vi "MicroGridExample.vi"() -> ()   [LabVIEW 2018]
uses:
  <vilib>/OPCUA/controls/NodeIds.ctl
  <vilib>/OPCUA/controls/NodeId.ctl
  <vilib>/OPCUA/client/Multiple Read Variant.vi
  GlobalVal.vi
  <vilib>/OPCUA/NI OPC UA Client.lvlib
panel:
  out "timestamp":timestamp
  out "OPCUA Server Error Log":errorcluster
  in  "Connect to Main Grid":bool
  out "Slide 8":u8(slide)
  out "Slide 7":u8(slide)
  out "Slide 6":u8(slide)
  out "Slide 5":u8(slide)
  out "Slide 4":u8(slide)
  out "Slide 2":u8(slide)
  out "Slide":u8(slide) scale=0.0..100.0
  out "Slide 3":u8(slide) scale=0.0..100.0
  out "Power":u8(slide) scale=0.0..100.0
  out "Power":u8(slide) scale=0.0..100.0
  in  "Tank":dbl(slide) scale=0.0..10.0
  in  "Photovoltaic":bool
  in  "Battery":bool
  out "Power":u8(slide) scale=0.0..100.0
  out "Power":u8(slide) scale=0.0..100.0
  out "Ki":dbl
  out "Kp":dbl
  out "tP":dbl
  out "kP":dbl
  in  "kP":dbl step=0.1
  in  "tf":dbl step=0.1
  out "tf":dbl
  out "kf":dbl
  in  "kf":dbl step=0.1
  in  "Ki":dbl step=0.1
  in  "Kp":dbl step=0.1
  in  "tP":dbl step=0.1
  in  "Program Stop":bool
  in  "Disconnect":bool
  in  "Connect Server":bool
  in  "OPC Server URL":string
  in  "Diesel 2":bool
  in  "Diesel 1":bool
  out "Device":string="PowerGenerator"
  in  "Solar irradiance":dbl(knob) scale=0.0..10.0
  in  "Load power":dbl(knob) scale=0.0..10.0
  in  "stop":bool
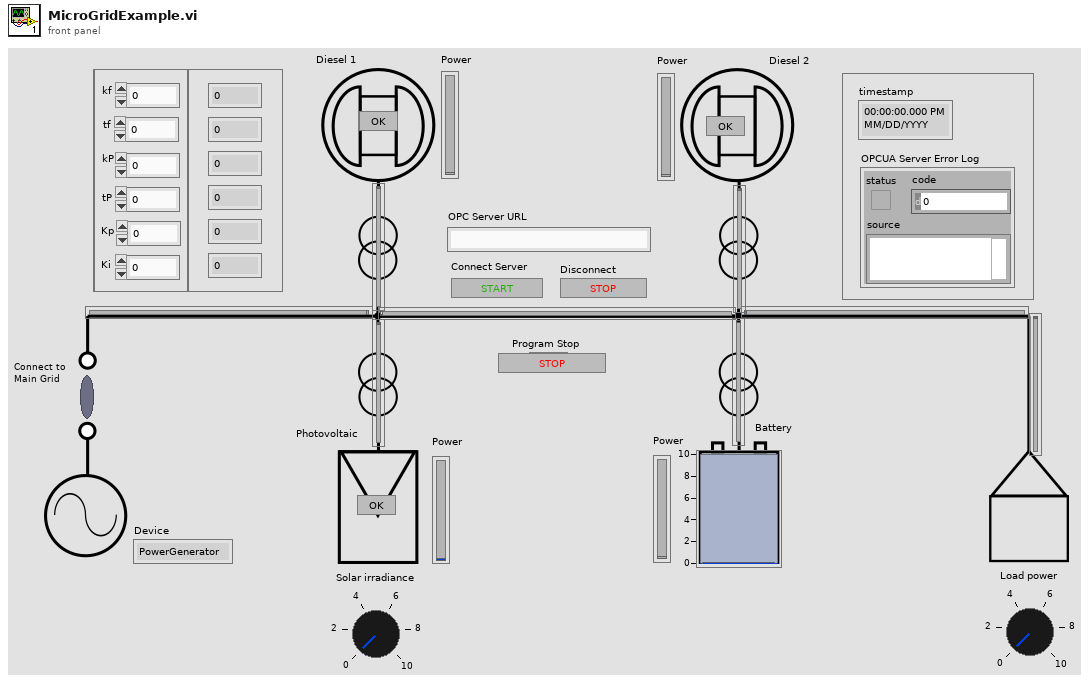
[diagram p1: front panel]
types:
  T1 = typedef "NodeIds.ctl" = T2[]
  T2 = typedef "NodeId.ctl" = string
  T3 = typedef "OPC UA Client Refnum.ctl" = refnum<k21>
  T4 = typedef "Read Variant Result.ctl" = cluster{"node ID":T2, "value ":variant, "timestamp":timestamp, "status":T5}
  T5 = typedef "OPC UA StatusCode.ctl" = u32
  T6 = enum32{"Invalid", "Standard", "Closed", "Hidden", "Minimized", "Maximized"}
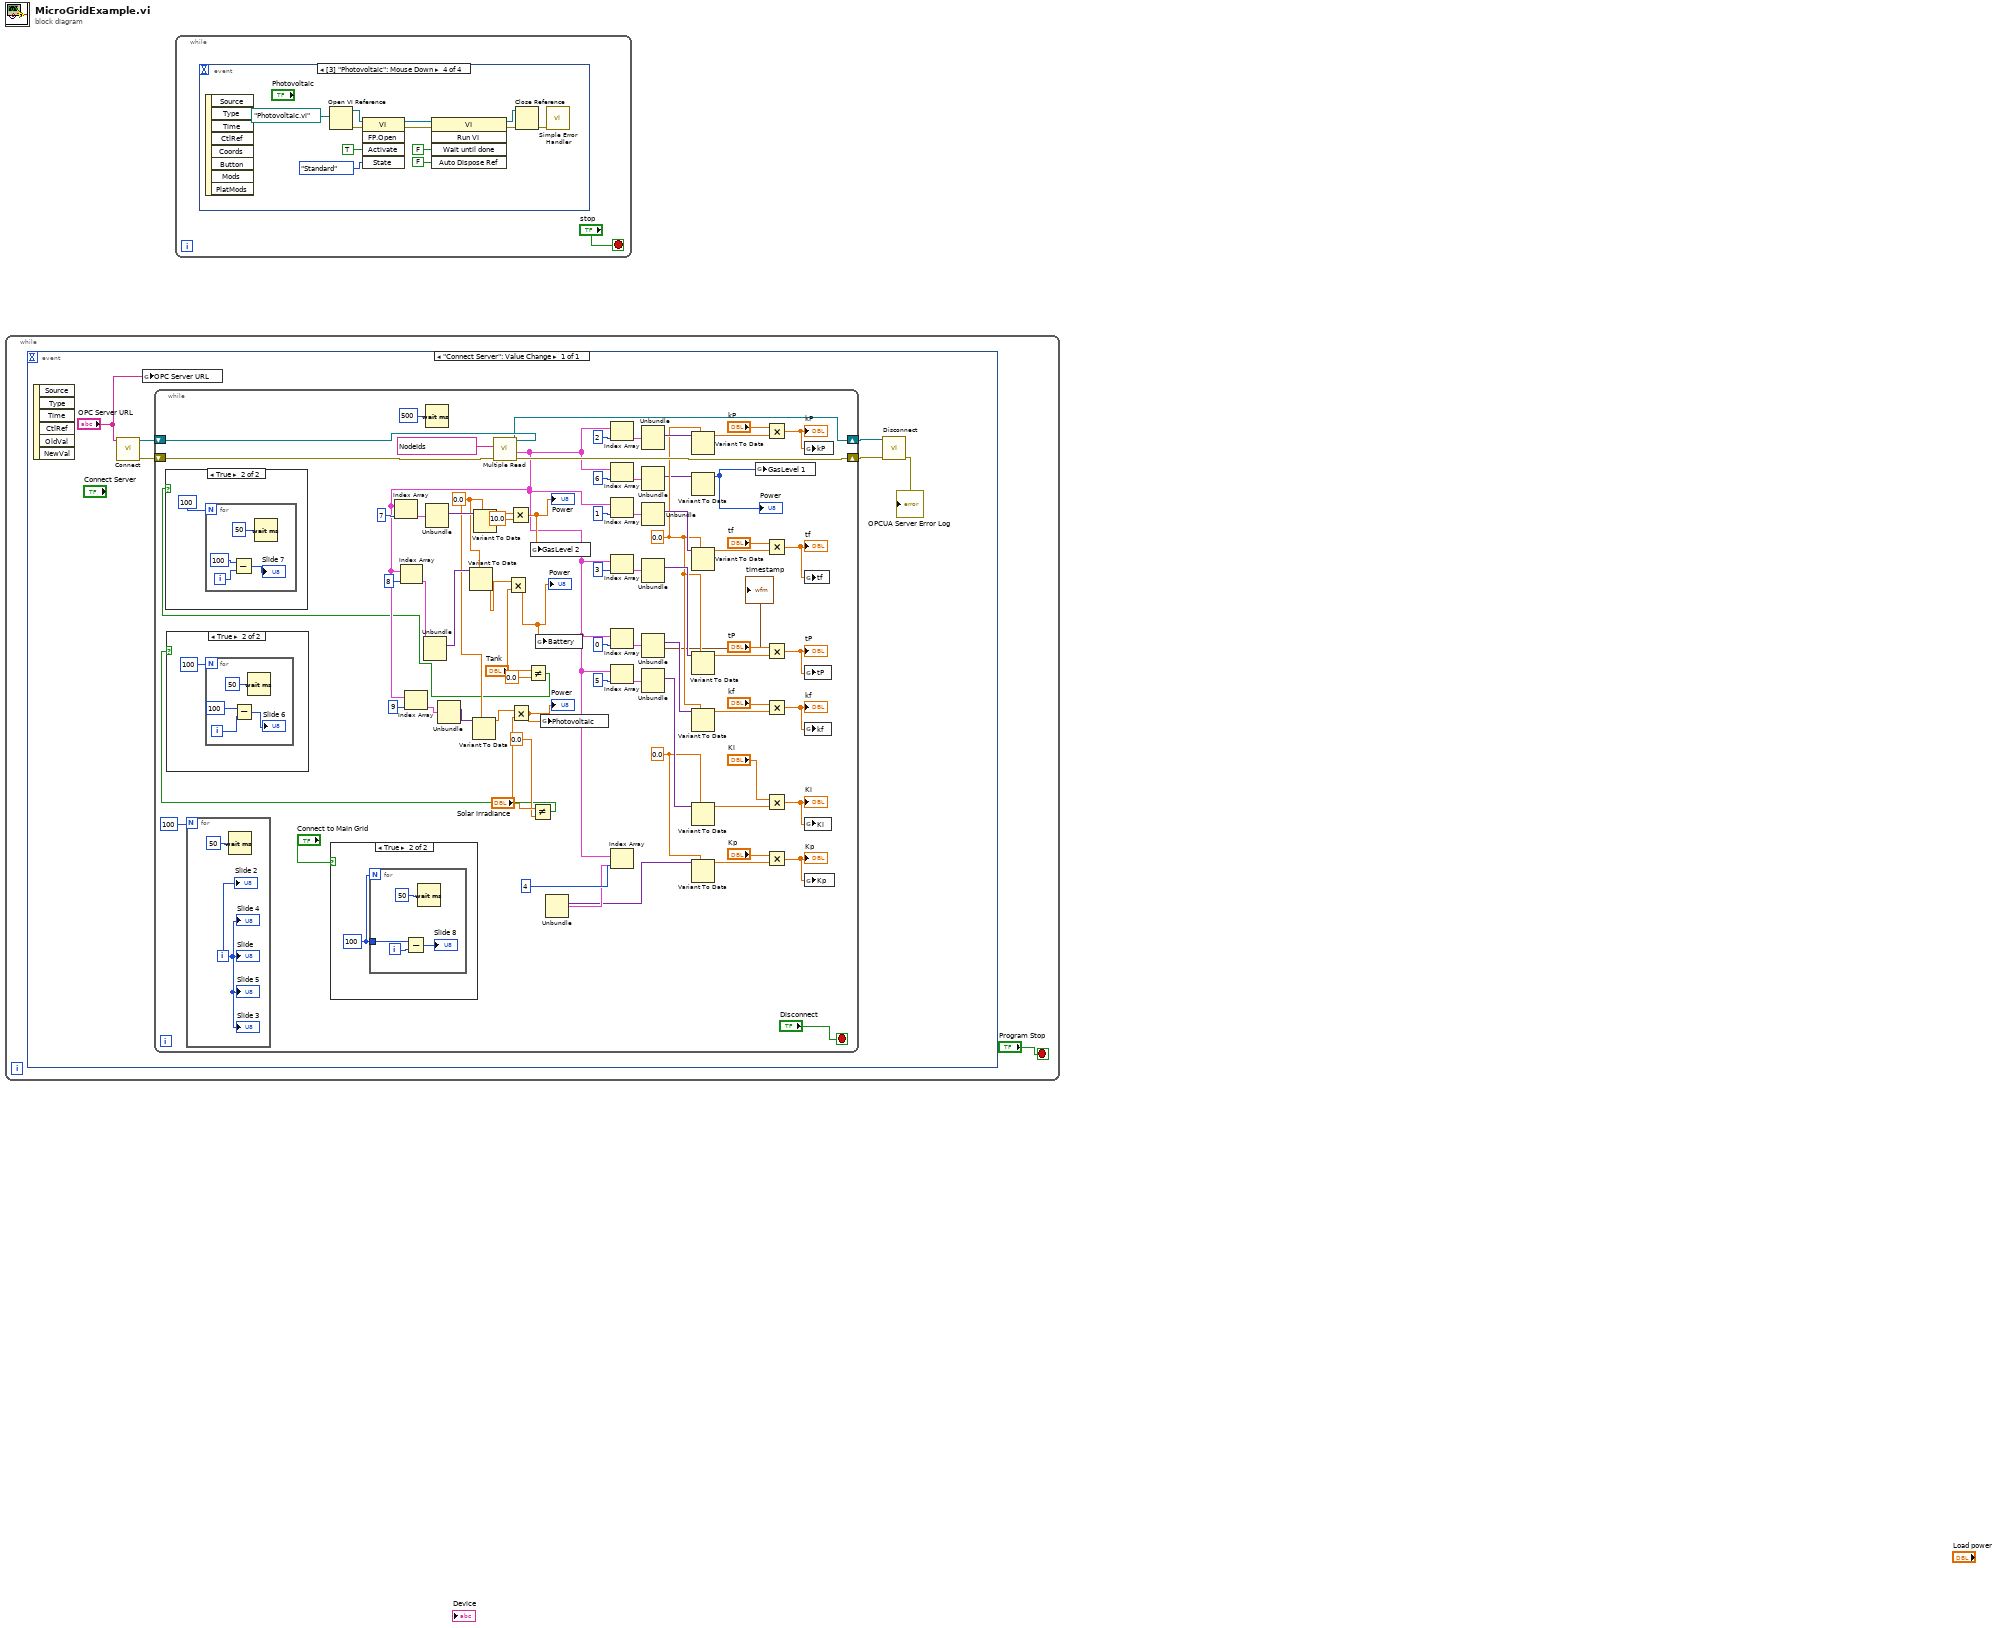
[diagram p0: block diagram]
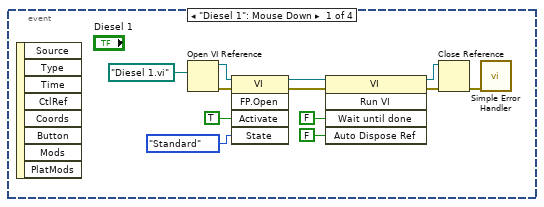
[diagram p2: hidden frame]
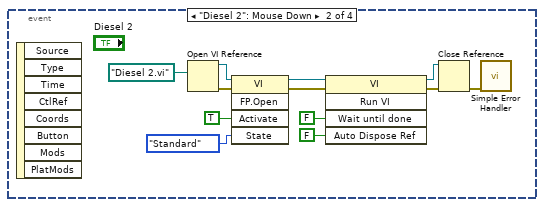
[diagram p3: hidden frame]
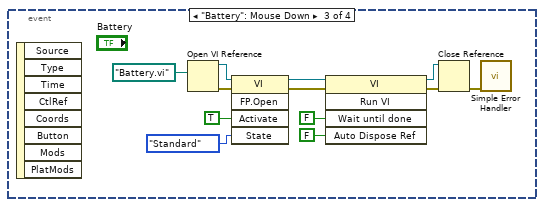
[diagram p4: hidden frame]
diagram:
  n1 = while {
    stop <- "Program Stop" stop-if-true
    n2 = event shown="[0] \"Connect Server\": Value Change" {
      selector: _ -> [_]
      dyn-events: _ -> [_]
      timeout: _ -> [_]
      event "Connect Server": Value Change {
        n3 = event-data() -> ()  [unwired: 1 in, 6 out]
        n4 = call <vilib>:"Connect.vi"("server endpoint URL"="OPC Server URL") -> ("error out"=w6:errorcluster, "OPC UA client refnum out"=w7:T3)  [unwired: 8 in, 1 out]
        n5 = global write "GlobalVal.vi" "OPC Server URL"("OPC Server URL") -> ()
        n6 = while {
          shift-right: [w80] -> w4
          shift-left: w7 -> [w83]
          shift-right: [w81] -> w5
          shift-left: w6 -> [w82]
          stop <- "Disconnect" stop-if-true
          w19 = 0.0
          w43 = 0.0
          w56 = 0.0
          n7 = for {
            N: 100 -> [_]
            i -> [w99]
            n8 = Wait (ms)(milliseconds to wait=u32 50) -> ()  [unwired: 1 out]
            "Slide 3" <- w99
            "Slide" <- w99
            "Slide 2" <- w99
            "Slide 4" <- w99
            "Slide 5" <- w99
          }
          n9 = case shown="True" "Connect to Main Grid" {
            frame False {
            }
            frame True {
              w84 = 100
              n10 = for {
                N: w84 -> [_]
                tunnel: w84 -> [w86]
                i -> [w85]
                n11 = Subtract(x=w86, y=w85) -> (x-y=→"Slide 8":i32)
                n12 = Wait (ms)(milliseconds to wait=u32 50) -> ()  [unwired: 1 out]
              }
            }
          }
          n13 = Wait (ms)(milliseconds to wait=u32 500) -> ()  [unwired: 1 out]
          n14 = call-poly <vilib>:"Multiple Read.vi"("error in (no error)"=w82, "node IDs"=T1 ["ns=2;i=8", "ns=2;i=9", "ns=2;i=10", "ns=2;i=11", "ns=2;i=12", "ns=2;i=13", "ns=2;i=2", "ns=3;i=2", "ns=4;i=2", "ns=5;i=2"], "OPC UA client refnum in"=w83) -> ("error out"=w81:errorcluster, "results"=w23:T4[], "OPC UA client refnum out"=w80:T3)  [unwired: 5 in, 1 out]
          n15 = Index Array(array=w23, index=7) -> (element=w33:T4)
          n16 = Index Array(array=w23, index=8) -> (element=w30:T4)
          n17 = Index Array(array=w23, index=9) -> (element=w21:T4)
          n18 = Unbundle(w30) -> ("value"=w29:variant)  [unwired: 3 out]
          n19 = Unbundle(w33) -> ("value"=w32:variant)  [unwired: 3 out]
          n20 = Unbundle(w21) -> ("value"=w20:variant)  [unwired: 3 out]
          n21 = Variant To Data(type=w19, Variant=w29) -> (data=w28:dbl)  [unwired: 1 in, 1 out]
          n22 = Variant To Data(type=w19, Variant=w20) -> (data=w18:dbl)  [unwired: 1 in, 1 out]
          n23 = Variant To Data(type=w19, Variant=w32) -> (data=w26:dbl)  [unwired: 1 in, 1 out]
          n24 = Multiply(x=w28, y="Tank") -> (x*y=w27:dbl)
          "Power" <- w27
          n25 = Multiply(x=w26, y=10.0) -> (x*y=w24:dbl)
          "Power" <- w24
          n26 = Multiply(x=w18, y="Solar irradiance") -> (x*y=w17:dbl)
          "Power" <- w17
          n27 = Not Equal?(x="Tank", y=0.0) -> (x != y?=w11:bool)
          n28 = case shown="True" w11 {
            frame False {
            }
            frame True {
              n29 = for {
                N: 100 -> [_]
                i -> [w92]
                n30 = Subtract(x=100, y=w92) -> (x-y=→"Slide 7":i32)
                n31 = Wait (ms)(milliseconds to wait=u32 50) -> ()  [unwired: 1 out]
              }
            }
          }
          n32 = global write "GlobalVal.vi" "GasLevel 2"(w24) -> ()
          n33 = Not Equal?(x="Solar irradiance", y=0.0) -> (x != y?=w14:bool)
          n34 = case shown="True" w14 {
            frame False {
            }
            frame True {
              n35 = for {
                N: 100 -> [_]
                i -> [w96]
                n36 = Subtract(x=100, y=w96) -> (x-y=→"Slide 6":i32)
                n37 = Wait (ms)(milliseconds to wait=u32 50) -> ()  [unwired: 1 out]
              }
            }
          }
          n38 = global write "GlobalVal.vi" "Battery"(w27) -> ()
          n39 = global write "GlobalVal.vi" "Photovoltaic"(w17) -> ()
          n40 = Index Array(array=w23, index=2) -> (element=w64:T4)
          n41 = Index Array(array=w23, index=6) -> (element=w38:T4)
          n42 = Index Array(array=w23, index=1) -> (element=w71:T4)
          n43 = Index Array(array=w23, index=3) -> (element=w58:T4)
          n44 = Index Array(array=w23, index=0) -> (element=w76:T4)
          n45 = Index Array(array=w23, index=5) -> (element=w45:T4)
          n46 = Index Array(array=w23, index=4) -> (element=w51:T4)
          n47 = Unbundle(w51) -> ("value"=w50:variant)  [unwired: 3 out]
          n48 = Unbundle(w64) -> ("value"=w63:variant)  [unwired: 3 out]
          n49 = Unbundle(w38) -> ("value"=w37:variant)  [unwired: 3 out]
          n50 = Unbundle(w71) -> ("value"=w70:variant)  [unwired: 3 out]
          n51 = Unbundle(w58) -> ("value"=w57:variant)  [unwired: 3 out]
          n52 = Unbundle(w76) -> ("value"=w75:variant, "timestamp"=→"timestamp":timestamp)  [unwired: 2 out]
          n53 = Unbundle(w45) -> ("value"=w44:variant)  [unwired: 3 out]
          n54 = Variant To Data(type=w56, Variant=w63) -> (data=w61:dbl)  [unwired: 1 in, 1 out]
          n55 = Variant To Data(Variant=w37) -> (data=w36:u8)  [unwired: 2 in, 1 out]
          "Power" <- w36
          n56 = Variant To Data(type=w56, Variant=w70) -> (data=w68:dbl)  [unwired: 1 in, 1 out]
          n57 = Variant To Data(type=w56, Variant=w57) -> (data=w54:dbl)  [unwired: 1 in, 1 out]
          n58 = Variant To Data(type=w56, Variant=w75) -> (data=w73:dbl)  [unwired: 1 in, 1 out]
          n59 = Variant To Data(type=w43, Variant=w44) -> (data=w42:dbl)  [unwired: 1 in, 1 out]
          n60 = Variant To Data(type=w43, Variant=w50) -> (data=w48:dbl)  [unwired: 1 in, 1 out]
          n61 = global write "GlobalVal.vi" "GasLevel 1"(w36) -> ()
          n62 = Multiply(x="kP", y=w61) -> (x*y=w60:dbl)
          "kP" <- w60
          n63 = Multiply(x="tf", y=w68) -> (x*y=w66:dbl)
          "tf" <- w66
          n64 = Multiply(x="tP", y=w54) -> (x*y=w53:dbl)
          "tP" <- w53
          n65 = Multiply(x="kf", y=w73) -> (x*y=w67:dbl)
          "kf" <- w67
          n66 = Multiply(x="Ki", y=w42) -> (x*y=w40:dbl)
          "Ki" <- w40
          n67 = Multiply(x="Kp", y=w48) -> (x*y=w47:dbl)
          "Kp" <- w47
          n68 = global write "GlobalVal.vi" "kP"(w60) -> ()
          n69 = global write "GlobalVal.vi" "tf"(w66) -> ()
          n70 = global write "GlobalVal.vi" "tP"(w53) -> ()
          n71 = global write "GlobalVal.vi" "kf"(w67) -> ()
          n72 = global write "GlobalVal.vi" "Ki"(w40) -> ()
          n73 = global write "GlobalVal.vi" "Kp"(w47) -> ()
        }
        n74 = call <vilib>:"Disconnect.vi"("error in (no error)"=w5, "OPC UA client refnum in"=w4) -> ("error out"=→"OPCUA Server Error Log":errorcluster)  [unwired: 9 in]
      }
    }
  }
  n75 = while {
    stop <- "stop" stop-if-true
    n76 = event shown="[3] \"Photovoltaic\": Mouse Down" {
      selector: _ -> [_ _ _ _]
      dyn-events: _ -> [_ _ _ _]
      timeout: _ -> [_ _ _ _]
      event "Diesel 1": Mouse Down {
        n77 = event-data() -> ()  [unwired: 1 in, 8 out]
        n78 = Open VI Reference(vi path=path "Diesel 1.vi") -> (vi reference=w113:refnum<vi>, error out=w112:errorcluster)  [unwired: 5 in]
        n79 = invoke class="VI" method="FP.Open"(reference=w113, error in=w112, "Activate"=TRUE ("Activate?"), "State"=T6."Standard") -> (reference out=w108:refnum<vi>, error out=w107:errorcluster)  [unwired: 1 in, 3 out]
        n80 = invoke class="VI" method="Run VI"(reference=w108, error in=w107, "Wait until done"=FALSE ("Wait Until Done"), "Auto Dispose Ref"=FALSE ("Auto Dispose Reference")) -> (reference out=w105:refnum<vi>, error out=w104:errorcluster)  [unwired: 1 in, 3 out]
        n81 = Close Reference(reference=w105, error in (no error)=w104) -> (error out=w106:errorcluster)
        n82 = call <vilib>:"Simple Error Handler.vi"("error in (no error)"=w106) -> ()  [unwired: 4 in, 5 out]
      }
      event "Diesel 2": Mouse Down {
        n83 = event-data() -> ()  [unwired: 1 in, 8 out]
        n84 = Open VI Reference(vi path=path "Diesel 2.vi") -> (vi reference=w119:refnum<vi>, error out=w120:errorcluster)  [unwired: 5 in]
        n85 = invoke class="VI" method="FP.Open"(reference=w119, error in=w120, "Activate"=TRUE ("Activate?"), "State"=T6."Standard") -> (reference out=w121:refnum<vi>, error out=w122:errorcluster)  [unwired: 1 in, 3 out]
        n86 = invoke class="VI" method="Run VI"(reference=w121, error in=w122, "Wait until done"=FALSE ("Wait Until Done"), "Auto Dispose Ref"=FALSE ("Auto Dispose Reference")) -> (reference out=w124:refnum<vi>, error out=w125:errorcluster)  [unwired: 1 in, 3 out]
        n87 = Close Reference(reference=w124, error in (no error)=w125) -> (error out=w123:errorcluster)
        n88 = call <vilib>:"Simple Error Handler.vi"("error in (no error)"=w123) -> ()  [unwired: 4 in, 5 out]
      }
      event "Battery": Mouse Down {
        n89 = event-data() -> ()  [unwired: 1 in, 8 out]
        n90 = Open VI Reference(vi path=path "Battery.vi") -> (vi reference=w131:refnum<vi>, error out=w132:errorcluster)  [unwired: 5 in]
        n91 = invoke class="VI" method="FP.Open"(reference=w131, error in=w132, "Activate"=TRUE ("Activate?"), "State"=T6."Standard") -> (reference out=w133:refnum<vi>, error out=w134:errorcluster)  [unwired: 1 in, 3 out]
        n92 = invoke class="VI" method="Run VI"(reference=w133, error in=w134, "Wait until done"=FALSE ("Wait Until Done"), "Auto Dispose Ref"=FALSE ("Auto Dispose Reference")) -> (reference out=w136:refnum<vi>, error out=w137:errorcluster)  [unwired: 1 in, 3 out]
        n93 = Close Reference(reference=w136, error in (no error)=w137) -> (error out=w135:errorcluster)
        n94 = call <vilib>:"Simple Error Handler.vi"("error in (no error)"=w135) -> ()  [unwired: 4 in, 5 out]
      }
      event "Photovoltaic": Mouse Down {
        n95 = event-data() -> ()  [unwired: 1 in, 8 out]
        n96 = Open VI Reference(vi path=path "Photovoltaic.vi") -> (vi reference=w143:refnum<vi>, error out=w144:errorcluster)  [unwired: 5 in]
        n97 = invoke class="VI" method="FP.Open"(reference=w143, error in=w144, "Activate"=TRUE ("Activate?"), "State"=T6."Standard") -> (reference out=w145:refnum<vi>, error out=w146:errorcluster)  [unwired: 1 in, 3 out]
        n98 = invoke class="VI" method="Run VI"(reference=w145, error in=w146, "Wait until done"=FALSE ("Wait Until Done"), "Auto Dispose Ref"=FALSE ("Auto Dispose Reference")) -> (reference out=w148:refnum<vi>, error out=w149:errorcluster)  [unwired: 1 in, 3 out]
        n99 = Close Reference(reference=w148, error in (no error)=w149) -> (error out=w147:errorcluster)
        n100 = call <vilib>:"Simple Error Handler.vi"("error in (no error)"=w147) -> ()  [unwired: 4 in, 5 out]
      }
    }
  }
